vi "CaculateSpotSize .vi"(0 "图像输入":T1, 1 "单个像元大小":dbl) -> (2 "光斑横向大小":dbl, 3 "光斑纵向大小":dbl, 4 "Image 2":T1(plugin-control))   [LabVIEW 2018]
uses:
  <vilib>/vision/Image Controls.llb/IMAQ Image.ctl
  <vilib>/vision/NI_Vision_Development_Module.lvlib
panel:
  out "Bounding Rect":T2
  out "纵向像素":dbl
  out "横向像素":dbl
  out "Image":T1(plugin-control)
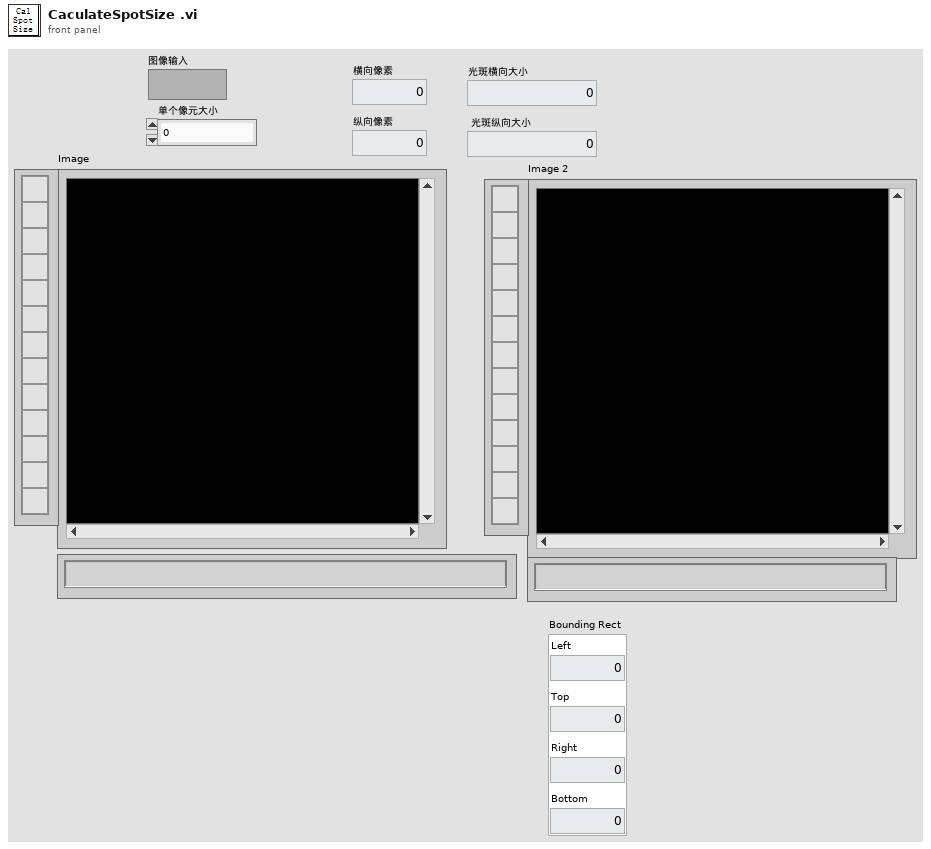
[diagram p1: front panel]
types:
  T1 = typedef "IMAQ Image.ctl" = refnum<image>
  T2 = cluster{"Left":dbl, "Top":dbl, "Right":dbl, "Bottom":dbl}
  T3 = typedef "Image Type" = u32
  T4 = enum32{"AutoM", "Close", "Dilate", "Erode", "Gradient", "Gradient out", "Gradient in", "Hit miss", "Open", "PClose", "POpen", "Thick", "Thin"}
  T5 = cluster{"Area":dbl, "Number of Holes":dbl, "Bounding Rect":cluster{"Left":dbl, "Top":dbl, "Right":dbl, "Bottom":dbl}, "Center of Mass":cluster{"X":dbl, "Y":dbl}, "Orientation":dbl, "Dimensions":cluster{"Width":dbl, "Height":dbl}}[]
  T6 = cluster{"Area":dbl, "Number of Holes":dbl, "Bounding Rect":cluster{"Left":dbl, "Top":dbl, "Right":dbl, "Bottom":dbl}, "Center of Mass":cluster{"X":dbl, "Y":dbl}, "Orientation":dbl, "Dimensions":cluster{"Width":dbl, "Height":dbl}}
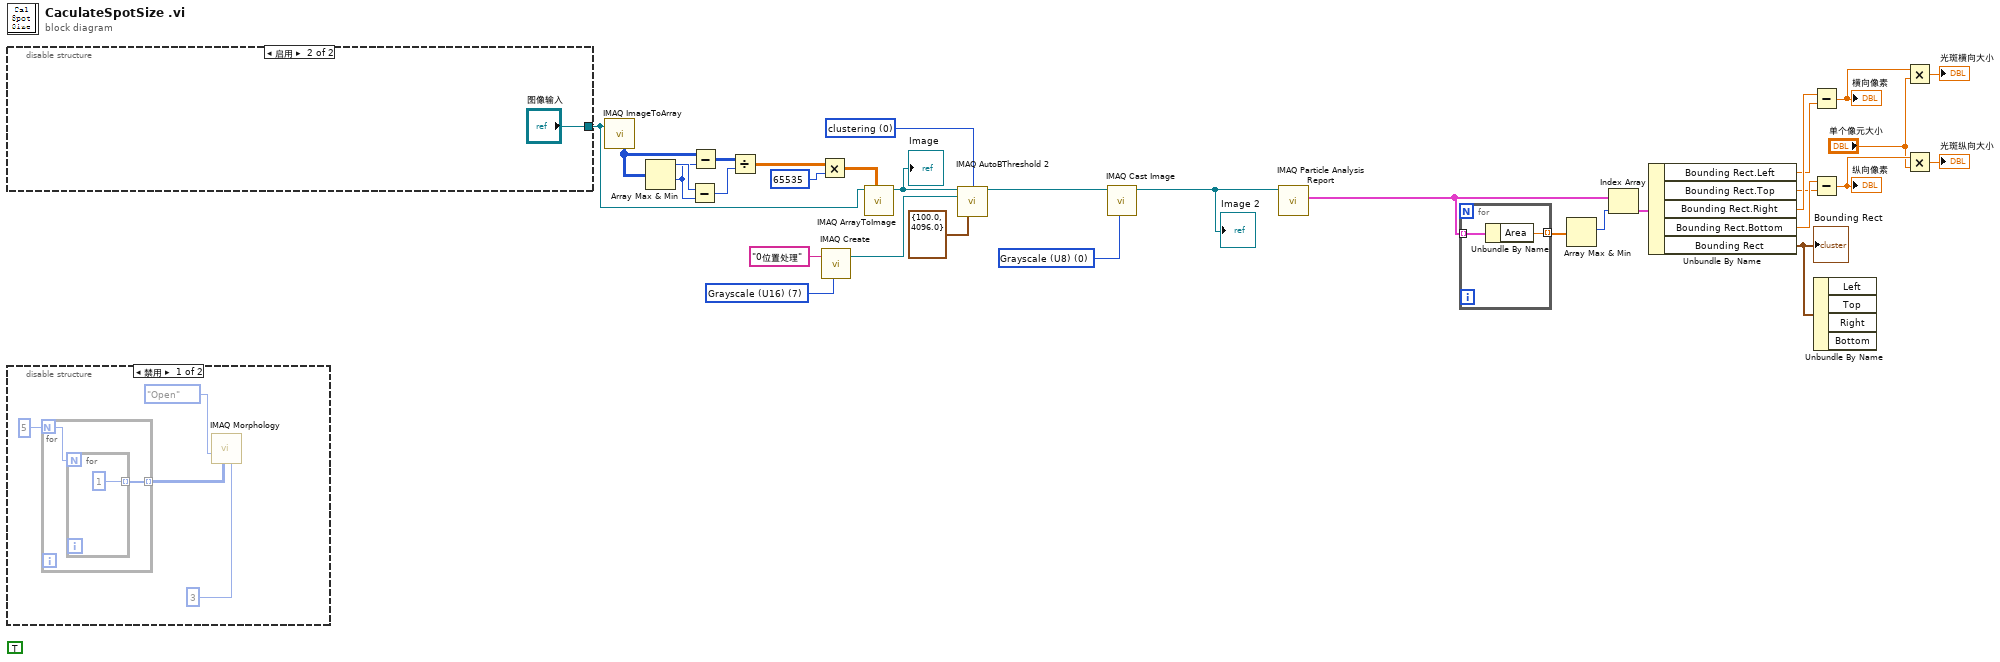
[diagram p0: block diagram]
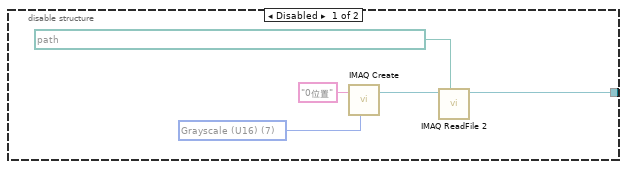
[diagram p3: hidden frame]
diagram:
  w2 = T3 0 items=["Grayscale (U8)", "Grayscale (I16)", "Grayscale (SGL)", "Complex (CSG)", "RGB (U32)", "HSL (U32)", "RGB (U64)", "Grayscale (U16)"] ("Image Type")
  w15 = T3 7 items=["Grayscale (U8)", "Grayscale (I16)", "Grayscale (SGL)", "Complex (CSG)", "RGB (U32)", "HSL (U32)", "RGB (U64)", "Grayscale (U16)"] ("Image Type")
  (unwired) TRUE ("Keep/Remove Particles (F)")
  w32 = 0 items=["clustering", "entropy", "metric", "moments", "inter-class variance"] ("Method (clustering)")
  n1 = disable-structure shown="启用" {
    disable-tunnel: [w34 "图像输入"] -> w5
    frame Disabled {
      w33 = T3 7 items=["Grayscale (U8)", "Grayscale (I16)", "Grayscale (SGL)", "Complex (CSG)", "RGB (U32)", "HSL (U32)", "RGB (U64)", "Grayscale (U16)"] ("Image Type")
      n2 = call "IMAQ Create"("Image Name"="0位置", "Image Type"=w33) -> ("New Image"=w36:T1)  [unwired: 3 in, 1 out]
      n3 = call "IMAQ ReadFile 2"("File Path"=path "E:/航天测量/软件/data/近远场数据/近场图/po123-456_发散角000.tiff", "Image"=w36) -> ("Image Out"=w34:T1)  [unwired: 5 in, 4 out]
    }
    frame Enabled {
    }
  }
  n4 = disable-structure shown="禁用" {
    frame Disabled {
      n5 = for {
        N: 5 -> [w44]
        tunnel: [w43] -> w39 mode=indexing
        n6 = for {
          N: w44 -> [_]
          tunnel: [1 ("Number of iterations (1)")] -> w43 mode=indexing
        }
      }
      n7 = call "IMAQ Morphology"("Number of iterations (1)"=3, "Structuring Element"=w39, "Operation"=T4."Open") -> ()  [unwired: 7 in, 2 out]
    }
    frame Enabled {
    }
  }
  n8 = call "IMAQ ImageToArray"("Image"=w5) -> ("Image Pixels (U16)"=w13:u16[][])  [unwired: 3 in, 4 out]
  n9 = Array Max & Min(array=w13) -> (max value=w11:u16, min value=w10:u16)  [unwired: 2 out]
  n10 = Subtract(x=w11, y=w10) -> (x-y=w9:u16)
  n11 = Subtract(x=w13, y=w10) -> (x-y=w12:u16[][])
  n12 = Divide(x=w12, y=w9) -> (x/y=w8:dbl[][])
  n13 = Multiply(x=w8, y=65535) -> (x*y=w4:dbl[][])
  n14 = call "IMAQ Create"("Image Name"="0位置处理", "Image Type"=w15) -> ("New Image"=w14:T1)  [unwired: 3 in, 1 out]
  n15 = call "IMAQ ArrayToImage"("Image Pixels (U16)"=w4, "Image"=w5) -> ("Image Out"=w6:T1)  [unwired: 8 in, 1 out]
  "Image" <- w6
  n16 = call "IMAQ AutoBThreshold 2"("Image Src"=w6, "Method (clustering)"=w32, "Image Dst"=w14, "Threshold Limits"=cluster{"Lower value":sgl, "Upper value":sgl} {"Lower value"=100.0, "Upper value"=4096.0}) -> ("Image Dst Out"=w31:T1)  [unwired: 9 in, 2 out]
  n17 = call "IMAQ Cast Image"("Image Type"=w2, "Image Src"=w31) -> ("Image Dst Out"=w3:T1)  [unwired: 8 in, 1 out]
  "Image 2" <- w3
  n18 = call "IMAQ Particle Analysis Report"("Image"=w3) -> ("Particle Reports (Pixels)"=w29:T5)  [unwired: 5 in, 5 out]
  n19 = for {
    tunnel: w29 -> [w47] mode=indexing
    tunnel: [w46] -> w30 mode=indexing
    n20 = Unbundle By Name(w47) -> ("Area"=w46:dbl)
  }
  n21 = Array Max & Min(array=w30) -> (max index (indices)=w28:i32)  [unwired: 3 out]
  n22 = Index Array(array=w29, index=w28) -> (element=w27:T6)
  n23 = Unbundle By Name(w27) -> ("Bounding Rect.Left"=w25:dbl, "Bounding Rect.Top"=w23:dbl, "Bounding Rect.Right"=w26:dbl, "Bounding Rect.Bottom"=w24:dbl, "Bounding Rect"=w1:T2)
  "Bounding Rect" <- w1
  n24 = Subtract(x=w26, y=w25) -> (x-y=w22:dbl)
  "横向像素" <- w22
  n25 = Subtract(x=w24, y=w23) -> (x-y=w20:dbl)
  "纵向像素" <- w20
  n26 = Unbundle By Name(w1) -> ()  [unwired: 4 out]
  n27 = Multiply(x=w22, y="单个像元大小") -> (x*y=→"光斑横向大小":dbl)
  n28 = Multiply(x=w20, y="单个像元大小") -> (x*y=→"光斑纵向大小":dbl)
